vi "read.vi"(8 "error in (no error)":errorcluster, 11 "Lesker Pressure in":refnum<class "Lesker Pressure.lvclass">) -> (0 "error out":errorcluster, 2 "Data":dbl[](array[numeric]), 3 "Lesker Pressure out":refnum<class "Lesker Pressure.lvclass">)   [LabVIEW 2024, in "Lesker Pressure.lvclass"]
uses:
  Lesker Pressure.lvclass
  Lesker Pressure.lvclass/Lesker Pressure.ctl
  Pressure Monitor.lvclass
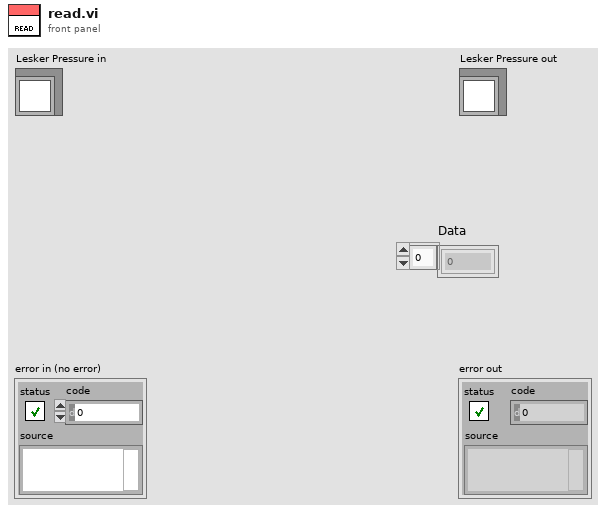
[diagram p1: front panel]
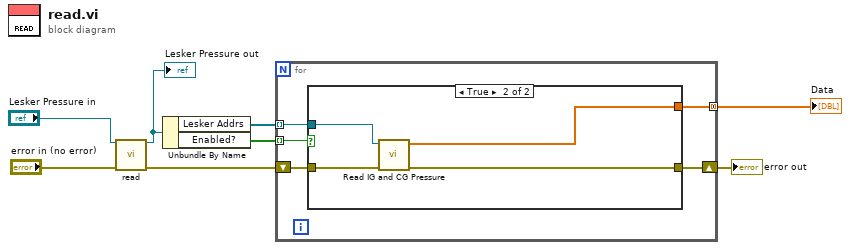
[diagram p0: block diagram]
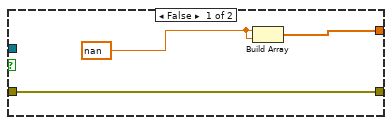
[diagram p2: hidden frame]
diagram:
  n1 = call-parent "read.vi"("error in (no error)"="error in (no error)", "Pressure Monitor in"="Lesker Pressure in") -> ("error out"=w6:errorcluster, "Pressure Monitor out"=w5:refnum<class "Lesker Pressure.lvclass">)  [unwired: 7 in, 1 out]
  "Lesker Pressure out" <- w5
  n2 = Unbundle By Name(w5) -> ("Lesker Addrs"=w3:refnum<visa-resource-name>[], "Enabled?"=w1:bool[])
  n3 = for {
    shift-right: [w12] -> w4
    shift-left: w6 -> [w13]
    tunnel: w3 -> [w11] mode=indexing
    tunnel: [w10] -> w2 mode=concatenating
    tunnel: w1 -> [w9] mode=indexing
    n4 = case shown="True" w9 {
      tunnel: w13 -> [w16 w20]
      tunnel: [w16 w18] -> w12
      tunnel: w11 -> [_ w19]
      tunnel: [w15 w17] -> w10
      frame False {
        w14 = nan ("Pressure")
        n5 = Build Array(w14, w14) -> (w15:dbl[])
      }
      frame True {
        n6 = call "Read IG and CG Pressure.vi"("error in (no error)"=w20, "VISA resource name"=w19) -> ("error out"=w18:errorcluster, "Data"=w17:dbl[])  [unwired: 8 in]
      }
    }
  }
  "error out" <- w4
  "Data" <- w2
